vi "ExecuteXML.vi"() -> ()   [LabVIEW 2017]
uses:
  RoutineData.vi
panel:
  in  "Boolean":bool
  out "XML String":string
  out "Routine Data":T1
  in  "Auto File Path":path=path "C:/Users/Bendethic/Desktop/AutoRoutineCreator/AutoFiles/1A.txt"
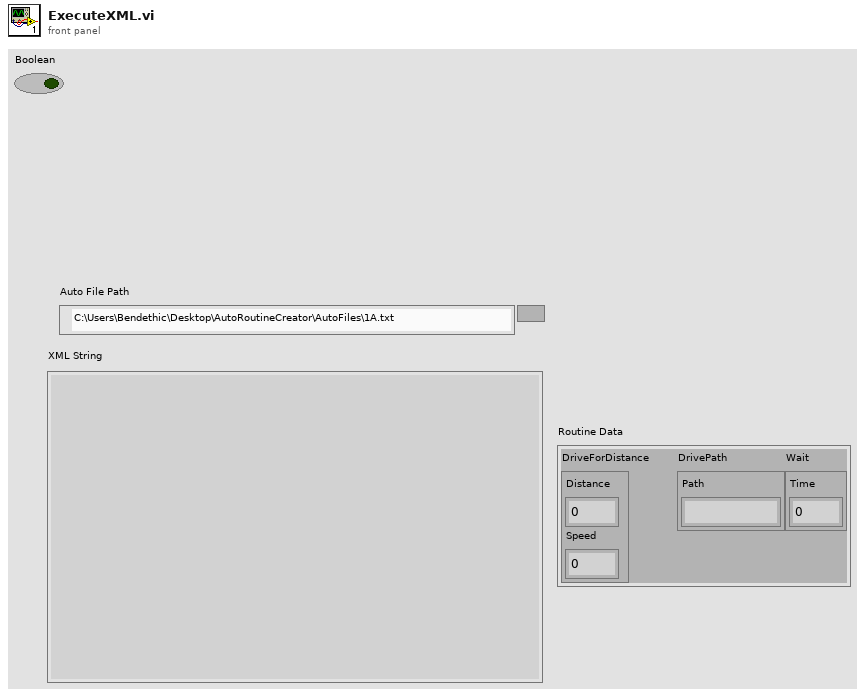
[diagram p1: front panel]
types:
  T1 = cluster{"DriveForDistance":cluster{"Distance":dbl, "Speed":dbl}, "DrivePath":cluster{"Path":string}, "Wait":cluster{"Time":u32}}
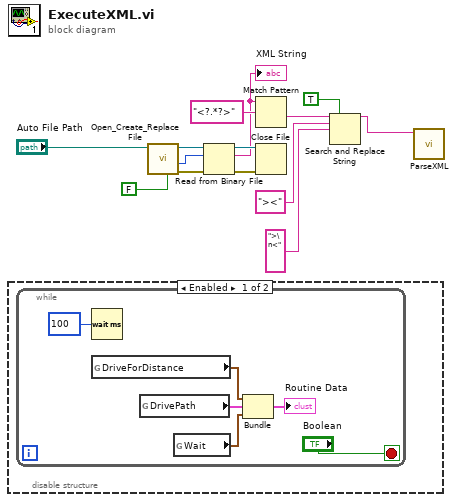
[diagram p0: block diagram]
diagram:
  n1 = disable-structure shown="Enabled" {
    frame Enabled {
      n2 = while {
        stop <- "Boolean" stop-if-true
        n3 = Wait (ms)(milliseconds to wait=u32 100) -> ()  [unwired: 1 out]
        n4 = global read "RoutineData.vi" "DriveForDistance"() -> (w19:cluster{"Distance":dbl, "Speed":dbl})
        n5 = global read "RoutineData.vi" "DrivePath"() -> (w18:cluster{"Path":string})
        n6 = global read "RoutineData.vi" "Wait"() -> (w17:cluster{"Time":u32})
        n7 = Bundle("DriveForDistance"=w19, "DrivePath"=w18, "Wait"=w17) -> (→"Routine Data":T1)  [unwired: 1 in]
      }
    }
    frame Disabled {
    }
  }
  n8 = call <vilib>:"Open_Create_Replace File.vi"("advisory dialog? (display:T)"=FALSE, "file path"="Auto File Path") -> ("error out"=w11:errorcluster, "file size (bytes)"=w13:i32, "refnum"=w9:refnum<file>)  [unwired: 6 in, 1 out]
  n9 = Read from Binary File(8:w11, 10:w13, 11:w9) -> (0:w12:errorcluster, 2:w7:string, 3:w10:refnum<file>)  [unwired: 3 in, 1 out]
  "XML String" <- w7
  n10 = Match Pattern(string=w7, regular expression="<?.*?>") -> (after substring=w4:string)  [unwired: 1 in, 3 out]
  n11 = Close File(refnum=w10, error in=w12) -> ()  [unwired: 2 out]
  n12 = Search and Replace String(replace all?=TRUE ("replace all? (F)"), input string=w4, search string="><", replace string=">\n<" ("replace string (\"\")")) -> (result string=w1:string)  [unwired: 4 in, 3 out]
  n13 = call "ParseXML.vi"("Node"=w1) -> ()  [unwired: 10 in, 1 out]
